vi "WSVCAP SHL Host LL I2C Write.vi"(0 "C1 Data Out [DUT Ordered]":u8[][](array[numeric]) format="%.0x", 1 "Wait Ticks":u32, 2 "Slave Address":u8, 5 "C2 Data Out [DUT Ordered]":u8[][](array[numeric]) format="%.0x", 7 "C3 Data Out [DUT Ordered]":u8[][](array[numeric]) format="%.0x", 9 "Socket Mask [U64]":u64=1 format="%016x", 11 "error in":errorcluster, 12 "Sub Address":u8=20, 13 "UUT Set (0/1)":u8, 14 "FPGA":T1) -> (10 "Status":u8[](array[numeric]), 15 "error out":errorcluster)   [LabVIEW 2012]
uses:
  Type Defs/WSVCAP SHL I2C FPGA Enum.ctl
  Type Defs/WSVCAP SHL Top Level Write Read State Enum.ctl
  Type Defs/WSVCAP SHL Transaction Enum.ctl
  Type Defs/WSVCAP SHL Top Level Control Enum.ctl
  Type Defs/WSVCAP SHL State.ctl
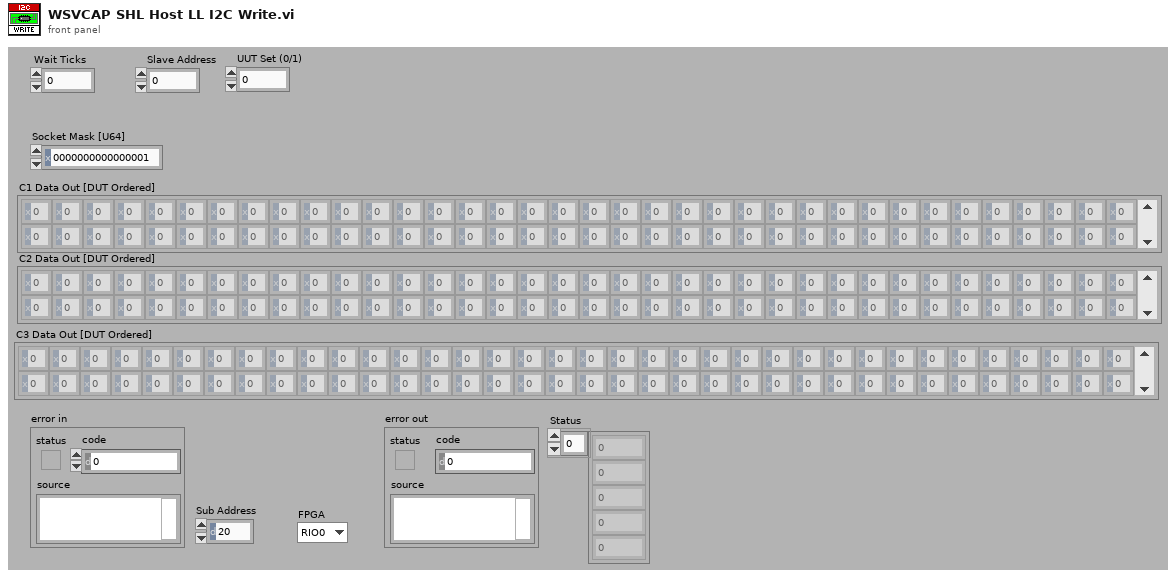
[diagram p1: front panel]
types:
  T1 = typedef "WSVCAP SHL I2C FPGA Enum.ctl" = enum16{"RIO0", "RIO1"}
  T2 = typedef "WSVCAP SHL Top Level Write Read State Enum.ctl" = enum16{"Start", "Write", "Read", "Get Status", "Wait Until Done"}
  T3 = typedef "WSVCAP SHL Top Level Control Enum.ctl" = enum16{"Start", "Cmd", "Transaction", "Wait Ticks", "Socket Mask", "UUT Set", "Slave Address", "Sub Address", "Bytes to Write", "Bytes to Read", "Write Data", "Write Flag", "Read Data", "Read Flag", "Ack Read", "Read Status Flag", "Ack Read Status", "Status", "Cycle Count", "Stop Cycle", "Exit"}
  T4 = typedef "WSVCAP SHL Transaction Enum.ctl" = enum16{"I2C-Read Data", "I2C-Write Data", "RFFE-Ext Write", "RFFE-Ext Read"}
  T5 = typedef "WSVCAP SHL State.ctl" = enum8{"Idle", "Transfer Data"}
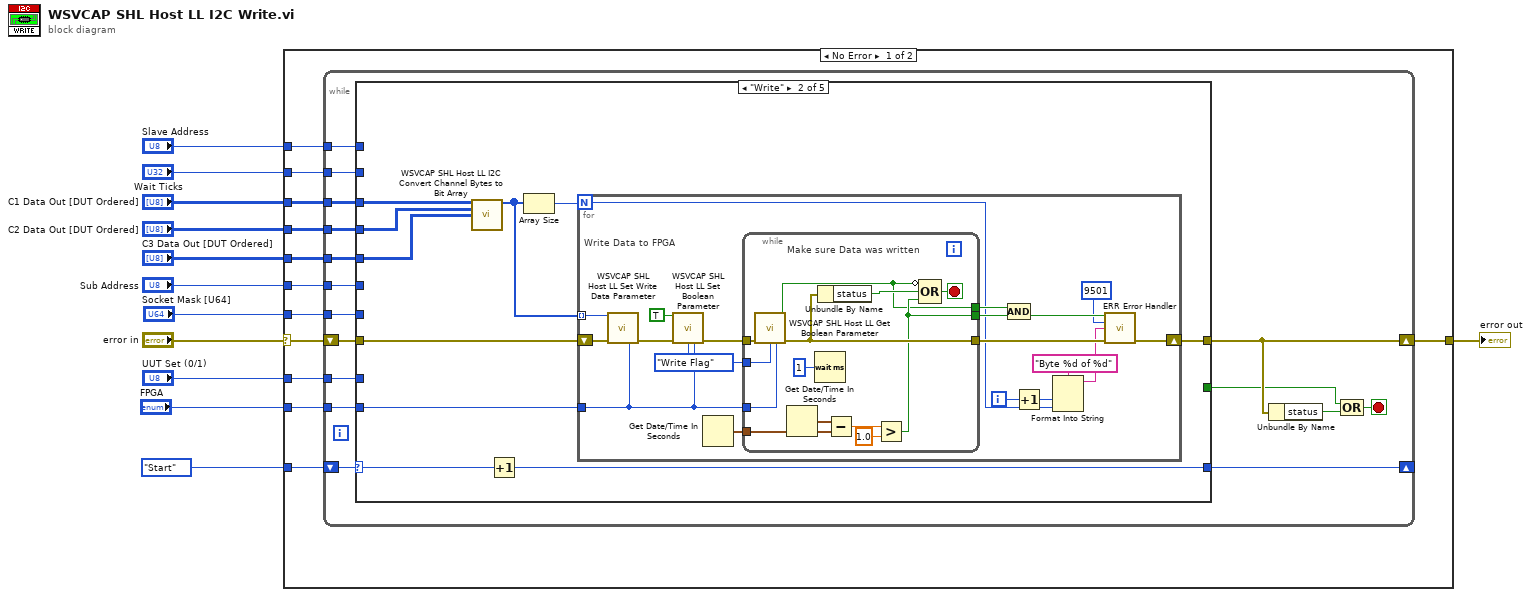
[diagram p0: block diagram]
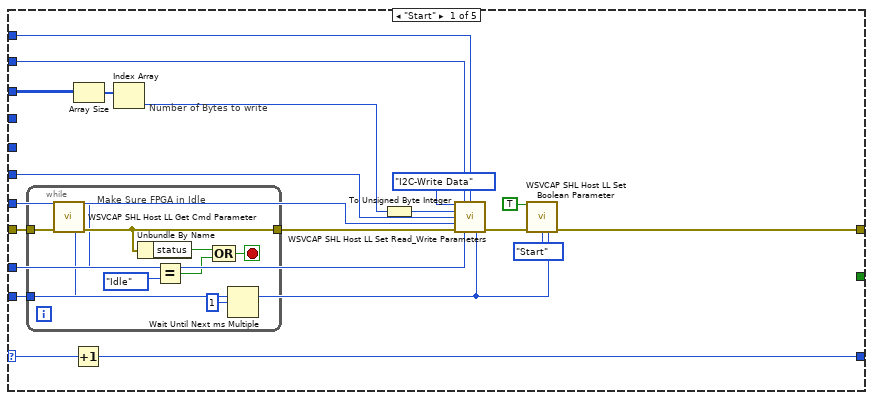
[diagram p2: hidden frame]
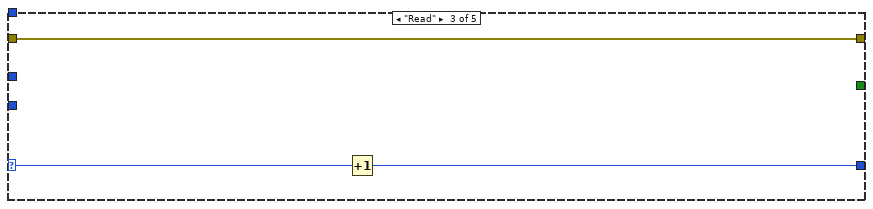
[diagram p3: hidden frame]
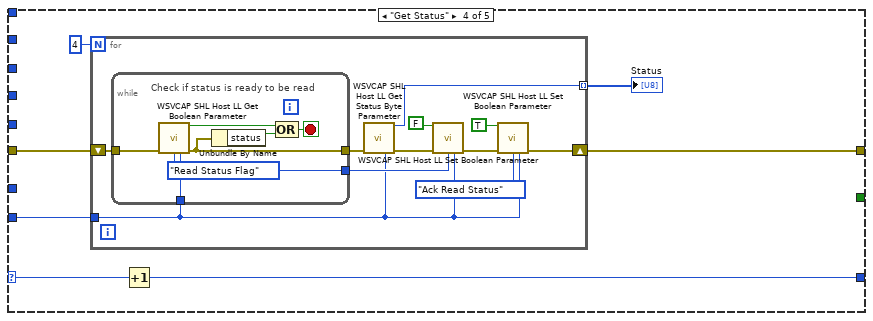
[diagram p4: hidden frame]
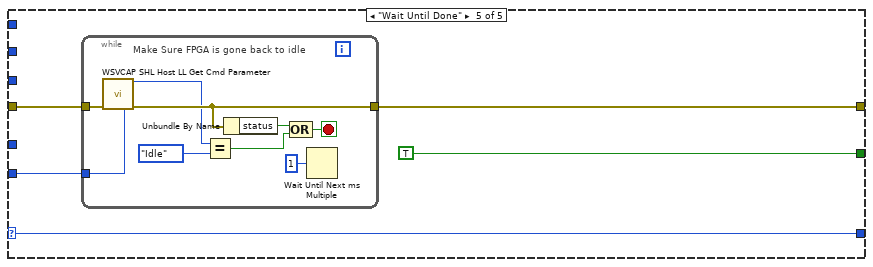
[diagram p5: hidden frame]
diagram:
  n1 = case shown="No Error" "error in" {
    selector: "error in" -> [w18 w152]
    tunnel: [w24 w152] -> w12
    tunnel: WSVCAP_SHL_Top_Level_Write_Read_State_Enum."Start" ("Write Read State") -> [w23 _]
    tunnel: "C1 Data Out [DUT Ordered]" -> [w22 _]
    tunnel: "C2 Data Out [DUT Ordered]" -> [w21 _]
    tunnel: "Sub Address" -> [w20 _]
    tunnel: "Socket Mask [U64]" -> [w19 _]
    tunnel: "Wait Ticks" -> [w17 _]
    tunnel: "C3 Data Out [DUT Ordered]" -> [w16 _]
    tunnel: "Slave Address" -> [w15 _]
    tunnel: "UUT Set (0/1)" -> [w14 _]
    tunnel: "FPGA" -> [w13 _]
    frame No Error {
      n2 = while {
        shift-right: [w39] -> w24
        shift-left: w18 -> [w40]
        shift-right: [w34] -> _
        shift-left: w23 -> [w35]
        tunnel: w22 -> [w33]
        tunnel: w21 -> [w32]
        tunnel: w20 -> [w31]
        tunnel: w19 -> [w30]
        tunnel: w17 -> [w29]
        tunnel: w16 -> [w28]
        tunnel: w15 -> [w27]
        tunnel: w14 -> [w26]
        tunnel: w13 -> [w25]
        stop <- w36 stop-if-true
        n3 = case shown="\"Write\"" w35 {
          selector: w35 -> [w57 w75 w111 w117 w140]
          tunnel: w40 -> [w58 w72 w112 w119 w142]
          tunnel: [w54 w77 w112 w118 w141] -> w39
          tunnel: [_ _ _ _ TRUE] -> w38
          tunnel: [w56 w76 w110 w116 w140] -> w34
          tunnel: w33 -> [w50 w71 _ _ _]
          tunnel: w32 -> [_ w70 _ _ _]
          tunnel: w31 -> [w46 _ _ _ _]
          tunnel: w30 -> [w45 _ _ _ _]
          tunnel: w29 -> [w44 _ _ _ _]
          tunnel: w28 -> [_ w69 _ _ _]
          tunnel: w27 -> [w43 _ _ _ _]
          tunnel: w26 -> [w42 _ _ _ _]
          tunnel: w25 -> [w41 w68 _ w113 w138]
          frame "Start" {
            # "Number of Bytes to write"
            n4 = while {
              tunnel: w58 -> [w63]
              tunnel: [w62] -> w55
              tunnel: w41 -> [w59]
              stop <- w67 stop-if-true
              # "Make Sure FPGA in Idle"
              n5 = call "WSVCAP SHL Host LL Get Cmd Parameter.vi"("error in (no error)"=w63, "FPGA"=w59) -> ("I2C_Cmd"=w61:T5, "error out"=w62:errorcluster)  [unwired: 12 in]
              n6 = Unbundle By Name(w62) -> ("status"=w60:bool)
              n7 = Equal?(x=w61, y=WSVCAP_SHL_State."Idle" ("Type")) -> (x = y?=w65:bool)
              n8 = Compound Arithmetic op=OR(w60, w65) -> (w67:bool)
              n9 = Wait Until Next ms Multiple(millisecond multiple=u32 1) -> ()  [unwired: 1 out]
            }
            n10 = Increment(x=w57) -> (x+1=w56:T2)
            n11 = Array Size(array=w50) -> (size(s)=w49:i32[])
            n12 = Index Array(array=w49) -> (element=w48:i32)  [unwired: 1 in]
            n13 = To Unsigned Byte Integer(number=w48) -> (unsigned 8bit integer=w47:u8)
            n14 = call "WSVCAP SHL Host LL Set Read_Write Parameters.vi"("Transaction"=WSVCAP_SHL_Transaction_Enum."I2C-Write Data", "Wait Ticks"=w44, "Slave Address"=w43, "Bytes"=w47, "Sub Address [U8]"=w46, "Socket Mask [U64]"=w45, "error in (no error)"=w55, "UUT Set (0/1)"=w42, "FPGA"=w41) -> ("error out"=w54:errorcluster)  [unwired: 6 in]
            n15 = call "WSVCAP SHL Host LL Set Boolean Parameter.vi"("Boolean In"=TRUE, "error in (no error)"=w54, "FPGA Top Level Control"=WSVCAP_SHL_Top_Level_Control_Enum."Start", "FPGA"=w41) -> ()  [unwired: 11 in, 1 out]
          }
          frame "Write" {
            # "Write Data to FPGA"
            n16 = call "WSVCAP SHL Host LL I2C Convert Channel Bytes to Bit Array.vi"("C1 Data Out"=w71, "C2 Data Out"=w70, "C3 Data Out"=w69) -> ("Write Data"=w73:u64[])  [unwired: 12 in]
            n17 = Increment(x=w75) -> (x+1=w76:T2)
            n18 = Array Size(array=w73) -> (size(s)=w74:i32)
            n19 = for {
              N: w74 -> [w80]
              shift-right: [w88] -> w77
              shift-left: w72 -> [w96]
              tunnel: w73 -> [w95] mode=indexing
              tunnel: w68 -> [w78]
              i -> [w83]
              w91 = WSVCAP_SHL_Top_Level_Control_Enum."Write Flag" ("FPGA Top Level Control")
              n20 = call "WSVCAP SHL Host LL Set Write Data Parameter.vi"("Write Byte In"=w95, "error in (no error)"=w96, "FPGA"=w78) -> ("error out"=w94:errorcluster)  [unwired: 12 in]
              n21 = call "WSVCAP SHL Host LL Set Boolean Parameter.vi"("Boolean In"=TRUE, "error in (no error)"=w94, "FPGA Top Level Control"=w91, "FPGA"=w78) -> ("error out"=w92:errorcluster)  [unwired: 11 in]
              n22 = Get Date/Time In Seconds() -> (seconds since 1Jan1904=w90:timestamp)
              n23 = while {
                tunnel: w92 -> [w107]
                tunnel: [w106] -> w89
                tunnel: w91 -> [w105]
                tunnel: w90 -> [w102]
                tunnel: [w99] -> w87
                tunnel: [w98] -> w86
                tunnel: w78 -> [w97]
                stop <- w109 stop-if-true
                # "Make sure Data was written"
                n24 = call "WSVCAP SHL Host LL Get Boolean Parameter.vi"("error in (no error)"=w107, "FPGA Top Level Control"=w105, "FPGA"=w97) -> ("Boolean Out"=w98:bool, "error out"=w106:errorcluster)  [unwired: 11 in]
                n25 = Get Date/Time In Seconds() -> (seconds since 1Jan1904=w103:timestamp)
                n26 = Wait (ms)(milliseconds to wait=u32 1) -> ()  [unwired: 1 out]
                n27 = Unbundle By Name(w106) -> ("status"=w104:bool)
                n28 = Subtract(x=w103, y=w102) -> (x-y=w101:dbl)
                n29 = Greater?(x=w101, y=1.0) -> (0:w99:bool)
                n30 = Compound Arithmetic op=OR(invert w98, w104, w99) -> (w109:bool)
              }
              n31 = Compound Arithmetic op=AND(w86, w87) -> (w85:bool)
              n32 = Increment(x=w83) -> (x+1=w79:i32)
              n33 = Format Into String(format string="Byte %d of %d", w79, w80) -> (resulting string=w82:string)  [unwired: 2 in, 1 out]
              n34 = call "ERR Error Handler.vi"("Error Status"=w85, "Error Code"=9501, "Cause Of Error"=w82, "Error In (no error)"=w89) -> ("Error Out"=w88:errorcluster)  [unwired: 11 in]
            }
          }
          frame "Read" {
            n35 = Increment(x=w111) -> (x+1=w110:T2)
          }
          frame "Get Status" {
            n36 = for {
              N: 4 -> [_]
              shift-right: [w129] -> w118
              shift-left: w119 -> [w130]
              tunnel: [w121] -> w114 mode=indexing
              tunnel: w113 -> [w120]
              n37 = while {
                tunnel: w130 -> [w135]
                tunnel: [w134] -> w128
                tunnel: [w132] -> w126
                tunnel: w120 -> [w131]
                stop <- w137 stop-if-true
                w132 = WSVCAP_SHL_Top_Level_Control_Enum."Read Status Flag" ("FPGA Top Level Control")
                # "Check if status is ready to be read"
                n38 = call "WSVCAP SHL Host LL Get Boolean Parameter.vi"("error in (no error)"=w135, "FPGA Top Level Control"=w132, "FPGA"=w131) -> ("Boolean Out"=w136:bool, "error out"=w134:errorcluster)  [unwired: 11 in]
                n39 = Unbundle By Name(w134) -> ("status"=w133:bool)
                n40 = Compound Arithmetic op=OR(w136, w133) -> (w137:bool)
              }
              n41 = call "WSVCAP SHL Host LL Get Status Byte Parameter.vi"("error in (no error)"=w128, "FPGA"=w120) -> ("I2C Status Byte"=w121:u8, "error out"=w127:errorcluster)  [unwired: 12 in]
              n42 = call "WSVCAP SHL Host LL Set Boolean Parameter.vi"("Boolean In"=FALSE ("Read Flag"), "error in (no error)"=w127, "FPGA Top Level Control"=w126, "FPGA"=w120) -> ("error out"=w122:errorcluster)  [unwired: 11 in]
              n43 = call "WSVCAP SHL Host LL Set Boolean Parameter.vi"("Boolean In"=TRUE ("Write Flag"), "error in (no error)"=w122, "FPGA Top Level Control"=WSVCAP_SHL_Top_Level_Control_Enum."Ack Read Status", "FPGA"=w120) -> ("error out"=w129:errorcluster)  [unwired: 11 in]
            }
            "Status" <- w114
            n44 = Increment(x=w117) -> (x+1=w116:T2)
          }
          frame "Wait Until Done" {
            n45 = while {
              tunnel: w142 -> [w146]
              tunnel: [w145] -> w141
              tunnel: w138 -> [w143]
              stop <- w148 stop-if-true
              # "Make Sure FPGA is gone back to idle"
              n46 = call "WSVCAP SHL Host LL Get Cmd Parameter.vi"("error in (no error)"=w146, "FPGA"=w143) -> ("I2C_Cmd"=w144:T5, "error out"=w145:errorcluster)  [unwired: 12 in]
              n47 = Equal?(x=w144, y=WSVCAP_SHL_State."Idle") -> (x = y?=w149:bool)
              n48 = Unbundle By Name(w145) -> ("status"=w150:bool)
              n49 = Compound Arithmetic op=OR(w150, w149) -> (w148:bool)
              n50 = Wait Until Next ms Multiple(millisecond multiple=u32 1) -> ()  [unwired: 1 out]
            }
          }
        }
        n51 = Unbundle By Name(w39) -> ("status"=w37:bool)
        n52 = Compound Arithmetic op=OR(w38, w37) -> (w36:bool)
      }
    }
    frame Error {
    }
  }
  "error out" <- w12
